vi "NI-USB-6210_Kernel.vi"() -> ()   [LabVIEW 2013]
uses:
  <vilib>/DAQmx/read.llb/DAQmx Read (Analog 2D DBL NChan NSamp).vi
  Global/measurementGlobal.vi
  <vilib>/DAQmx/configure/timing.llb/DAQmx Timing (Sample Clock).vi
  <vilib>/DAQmx/create/channels.llb/DAQmx Create Channel (AI-Voltage-Basic).vi
  <vilib>/DAQmx/miscellaneous.llb/DAQmx Fill In Error Info.vi
panel:
  out "element":i32
  out "data":dbl[][](array[numeric]) format="%0.2f"
  out "Input No of samples":i32
  out "Cases":string[](array[string])
  out "error out":errorcluster
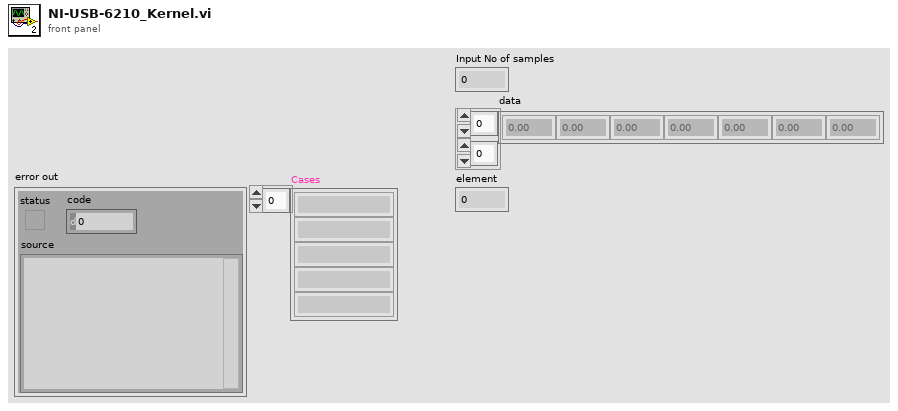
[diagram p1: front panel]
types:
  T1 = cluster{"Chan No":i32, "Low Volt Limit (-10V)":dbl, "High Volt Limit (10V)":dbl}[]
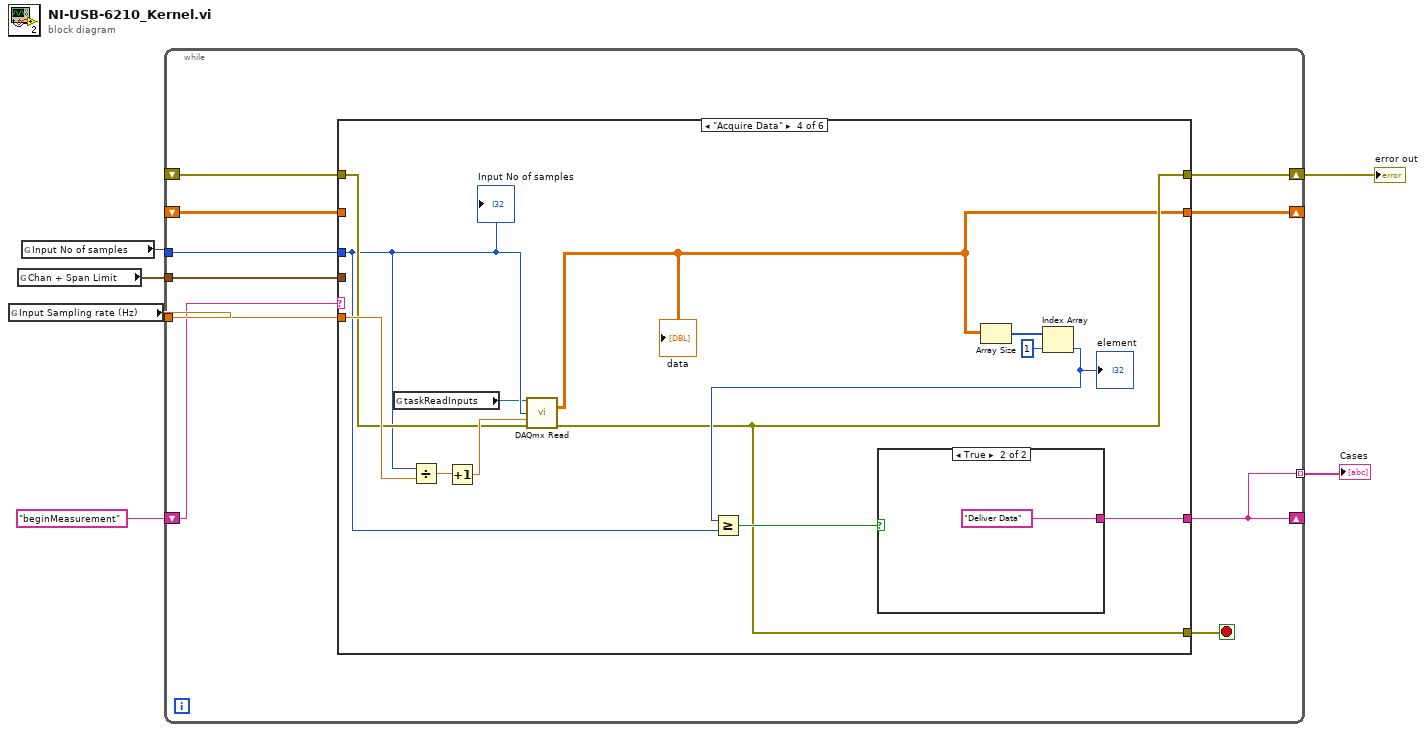
[diagram p0: block diagram]
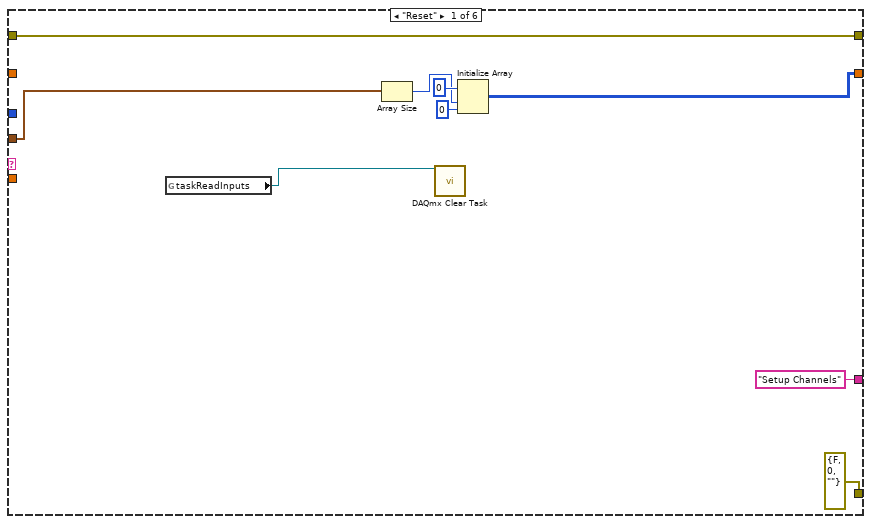
[diagram p2: hidden frame]
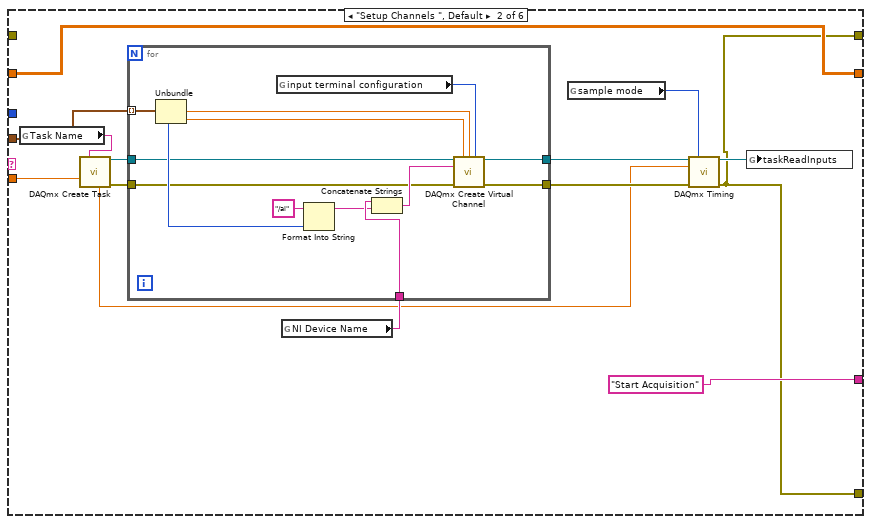
[diagram p3: hidden frame]
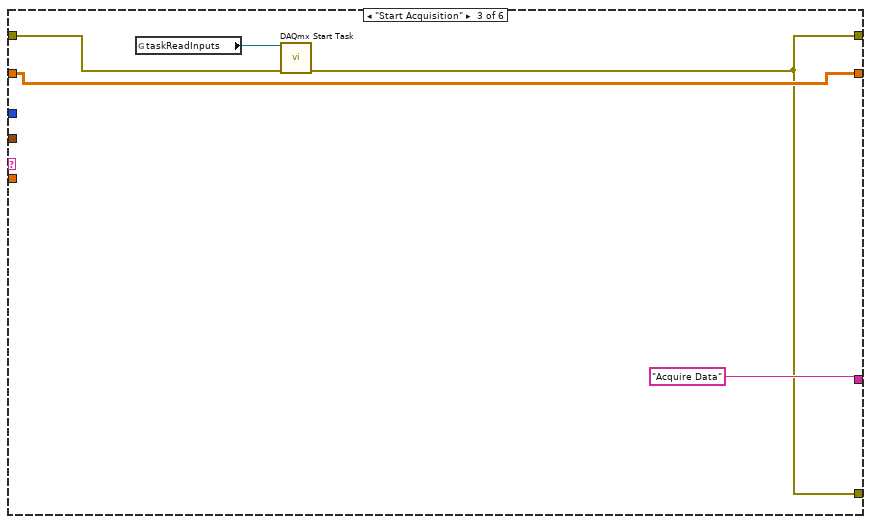
[diagram p4: hidden frame]
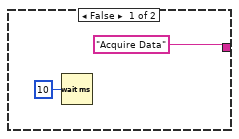
[diagram p5: hidden frame]
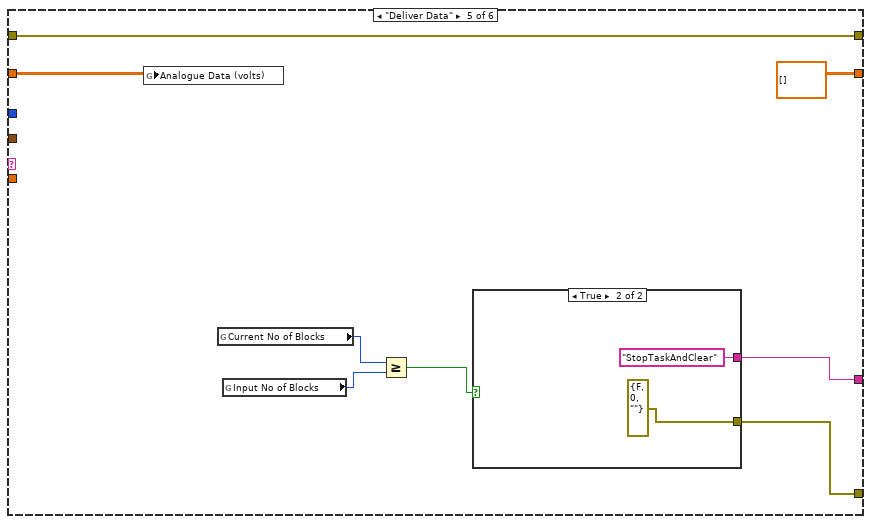
[diagram p6: hidden frame]
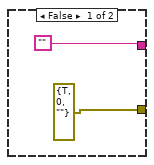
[diagram p7: hidden frame]
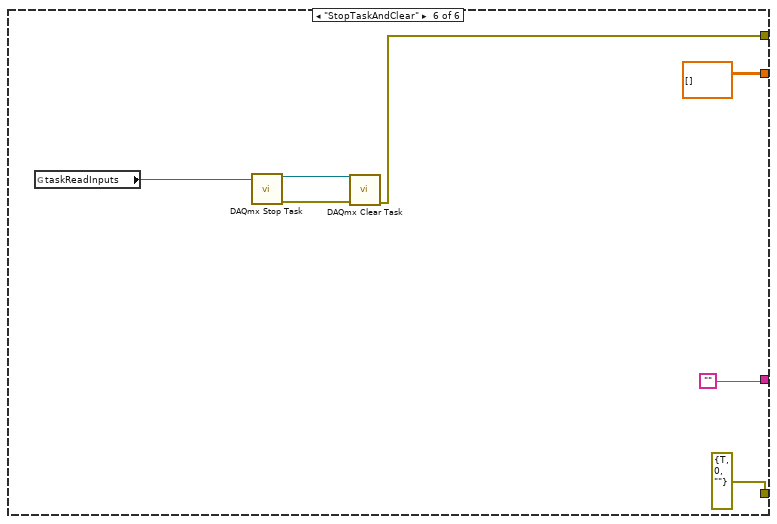
[diagram p8: hidden frame]
diagram:
  n1 = global read "measurementGlobal.vi" "Input Sampling rate (Hz)"() -> (w5:dbl)
  n2 = global read "measurementGlobal.vi" "Chan + Span Limit"() -> (w1:T1)
  n3 = global read "measurementGlobal.vi" "Input No of samples"() -> (w6:i32)
  n4 = while {
    tunnel: w6 -> [w16]
    tunnel: w5 -> [w15]
    shift-right: [w14] -> w4
    shift-left: _ -> [w13]
    shift-right: [w11] -> _
    shift-left: _ -> [w10]
    shift-right: [w8] -> _
    shift-left: "beginMeasurement" -> [w9]
    tunnel: [w8] -> w2 mode=indexing
    tunnel: w1 -> [w7]
    stop <- w12 stop-if-true
    n5 = case shown="\"Acquire Data\"" w9 {
      tunnel: w16 -> [_ _ _ w63 _ _]
      tunnel: w15 -> [_ w34 _ w69 _ _]
      tunnel: [w23 w29 w52 w59 w80 w89] -> w14
      tunnel: w13 -> [w23 _ w55 w66 w80 _]
      tunnel: [errorcluster {"status"=FALSE, "code"=0, "source"=""} ("error out") w29 w52 w59 w76 errorcluster {"status"=TRUE, "code"=0, "source"=""} ("error out")] -> w12
      tunnel: [w18 w32 w54 w57 dbl[][] [] ("data") dbl[][] [] ("data")] -> w11
      tunnel: w10 -> [_ w32 w54 _ w74 _]
      tunnel: ["Setup Channels" "Start Acquisition" "Acquire Data" w60 w75 ""] -> w8
      tunnel: w7 -> [w22 w38 _ _ _ _]
      frame "Reset" {
        n6 = global read "measurementGlobal.vi" "taskReadInputs"() -> (w17:refnum<k21>)
        n7 = Array Size(array=w22) -> (size(s)=w19:i32)
        n8 = call <vilib>:"DAQmx Clear Task.vi"("task in"=w17) -> ()  [unwired: 14 in, 1 out]
        n9 = Initialize Array(0 ("dimension size"), w19, 0 ("dimension size")) -> (w18:i32[][])
      }
      frame "Setup Channels ", Default {
        n10 = global read "measurementGlobal.vi" "Task Name"() -> (w26:string)
        n11 = call <vilib>:"DAQmx Create Task.vi"("new task name"=w26) -> ("task out"=w28:refnum<k21>, "error out"=w27:errorcluster)  [unwired: 13 in]
        n12 = global read "measurementGlobal.vi" "NI Device Name"() -> (w37:string)
        n13 = for {
          tunnel: w38 -> [w51] mode=indexing
          tunnel: w37 -> [w46]
          tunnel: [w43] -> w36
          tunnel: [w42] -> w35
          tunnel: w28 -> [w40]
          tunnel: w27 -> [w39]
          n14 = Unbundle(w51) -> ("Chan No"=w48:i32, "Low Volt Limit (-10V)"=w50:dbl, "High Volt Limit (10V)"=w49:dbl)
          n15 = global read "measurementGlobal.vi" "input terminal configuration"() -> (w41:i32)
          n16 = Format Into String(initial string="/ai", w48) -> (resulting string=w45:string)  [unwired: 2 in, 1 out]
          n17 = Concatenate Strings(w46, w45) -> (w44:string)
          n18 = call-poly <vilib>:"DAQmx Create Virtual Channel.vi"("task in"=w40, "maximum value"=w49, "minimum value"=w50, "input terminal configuration"=w41, "physical channels"=w44, "error in"=w39) -> ("task out"=w43:refnum<k21>, "error out"=w42:errorcluster)  [unwired: 8 in]
        }
        n19 = global read "measurementGlobal.vi" "sample mode"() -> (w33:i32)
        n20 = call-poly <vilib>:"DAQmx Timing.vi"("task/channels in"=w36, "sample mode"=w33, "rate"=w34, "error in"=w35) -> ("task out"=w31:refnum<k21>, "error out"=w29:errorcluster)  [unwired: 10 in]
        n21 = global write "measurementGlobal.vi" "taskReadInputs"(w31) -> ()
      }
      frame "Start Acquisition" {
        n22 = global read "measurementGlobal.vi" "taskReadInputs"() -> (w56:refnum<k21>)
        n23 = call <vilib>:"DAQmx Start Task.vi"("task/channels in"=w56, "error in"=w55) -> ("error out"=w52:errorcluster)  [unwired: 12 in, 1 out]
      }
      frame "Acquire Data" {
        n24 = global read "measurementGlobal.vi" "taskReadInputs"() -> (w58:refnum<k21>)
        n25 = Divide(x=w63, y=w69) -> (x/y=w68:dbl)
        n26 = Increment(x=w68) -> (x+1=w67:dbl)
        n27 = call-poly <vilib>:"DAQmx Read.vi"("task/channels in"=w58, "number of samples per channel"=w63, "timeout"=w67, "error in"=w66) -> ("data"=w57:dbl[][], "error out"=w59:errorcluster)  [unwired: 9 in, 1 out]
        "data" <- w57
        n28 = Array Size(array=w57) -> (size(s)=w65:i32[])
        n29 = Index Array(array=w65, index=1) -> (element=w62:i32)
        "element" <- w62
        n30 = Greater Or Equal?(x=w62, y=w63) -> (x >= y?=w61:bool)
        n31 = case shown="True" w61 {
          tunnel: ["Acquire Data" "Deliver Data"] -> w60
          frame False {
            n32 = Wait (ms)(milliseconds to wait=u32 10) -> ()  [unwired: 1 out]
          }
          frame True {
          }
        }
        "Input No of samples" <- w63
      }
      frame "Deliver Data" {
        n33 = global write "measurementGlobal.vi" "Analogue Data (volts)"(w74) -> ()
        n34 = global read "measurementGlobal.vi" "Current No of Blocks"() -> (w79:i32)
        n35 = global read "measurementGlobal.vi" "Input No of Blocks"() -> (w78:i32)
        n36 = Greater Or Equal?(x=w79, y=w78) -> (x >= y?=w77:bool)
        n37 = case shown="True" w77 {
          tunnel: [errorcluster {"status"=TRUE, "code"=0, "source"=""} ("error out") errorcluster {"status"=FALSE, "code"=0, "source"=""} ("error out")] -> w76
          tunnel: ["" "StopTaskAndClear"] -> w75
          frame False {
          }
          frame True {
          }
        }
      }
      frame "StopTaskAndClear" {
        n38 = global read "measurementGlobal.vi" "taskReadInputs"() -> (w91:refnum<k21>)
        n39 = call <vilib>:"DAQmx Stop Task.vi"("task/channels in"=w91) -> ("task out"=w88:refnum<k21>, "error out"=w90:errorcluster)  [unwired: 13 in]
        n40 = call <vilib>:"DAQmx Clear Task.vi"("task in"=w88, "error in"=w90) -> ("error out"=w89:errorcluster)  [unwired: 13 in]
      }
    }
  }
  "error out" <- w4
  "Cases" <- w2
